vi "HapticSTM_Feedblackless_testdata.vi"() -> ()   [LabVIEW 2017]
uses:
  <userlib>/HapticSTM/Feedbackless - Testdata/Project/feedbackless.lvproj/HapticSTM.lvlib
  <userlib>/HapticSTM/Feedbackless - Testdata/Project/feedbackless.lvproj/GlobalClicksHeight.vi
  <vilib>/ptbypt/NI_PtbyPt.lvlib
  <vilib>/Utility/file.llb/Read Delimited Spreadsheet (DBL).vi
  <vilib>/Analysis/3filter.llb/Filter Passband Type.ctl
  <vilib>/Analysis/NI_AALBase.lvlib
panel:
  in  "Force Mode":u16(ring) items=["Stacked Logs", "Simple Log", "Linear"]
  out "Button":bool
  out "Zpos":cluster{dbl, "Y":dbl, i16}(graph)
  out "Filtered Current":dbl
  in  "Reset Clicks":bool
  out "Scaled Force and Current":cluster{dbl, "Filtered x":dbl, dbl}(graph)
  in  "Maximum (pA)":dbl=9000.0
  in  "Setpoint (pA)":dbl=100.0
  out "PLANE HEIGHT":dbl
  out "Current":dbl
  out "Origin Y":dbl
  out "Origin X":dbl
  out "Output Z":dbl
  in  "Rough adjust":dbl
  out "Nano Z":dbl
  out "Width":dbl
  out "VY":dbl
  out "VZ":dbl
  out "VX":dbl
  in  "Drag":dbl=1.0
  in  "STOP":bool
  in  "START":bool
  out "Fy":dbl
  out "Fz":dbl
  out "phi":dbl
  out "psi":dbl
  out "Fx":dbl
  out "theta":dbl
  out "x":dbl
  out "y":dbl
  out "z":dbl
  in  "Fine adjust":dbl=3.5
  out "Clicks":dbl
  out "Height":dbl
  # "Sample Window"
  # "Position"
  # "Sensitivity"
  # "Force"
  # "STM I/O"
  # "Angles"
  # "Current"
  # "Velocity"
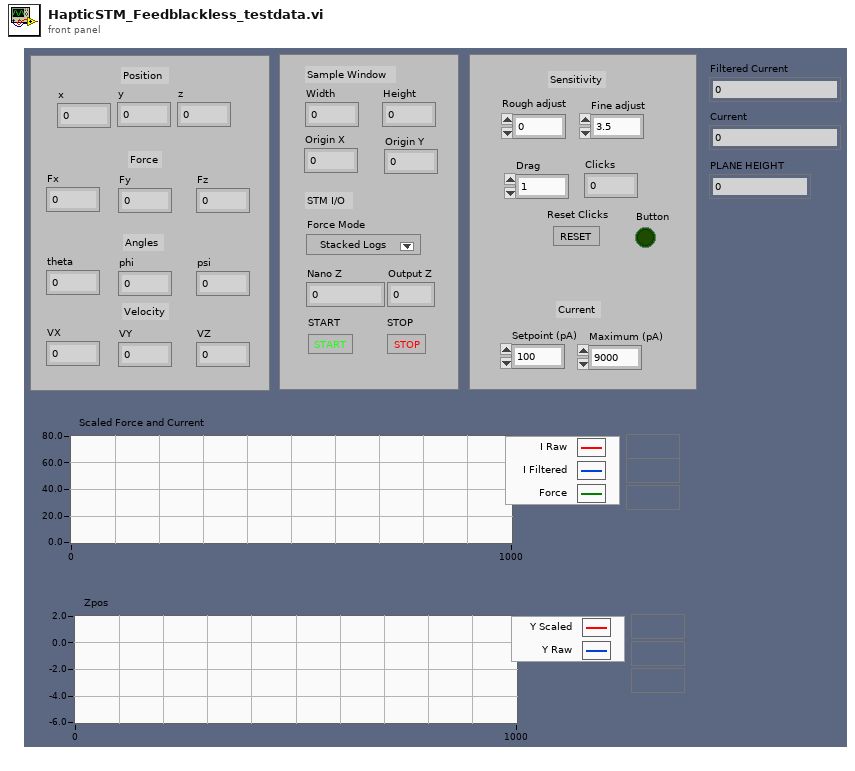
[diagram p1: front panel]
types:
  T1 = typedef "NI_AALBase.lvlib/Filter Passband Type.ctl" = enum32{"Lowpass", "Highpass", "Bandpass", "Bandstop"}
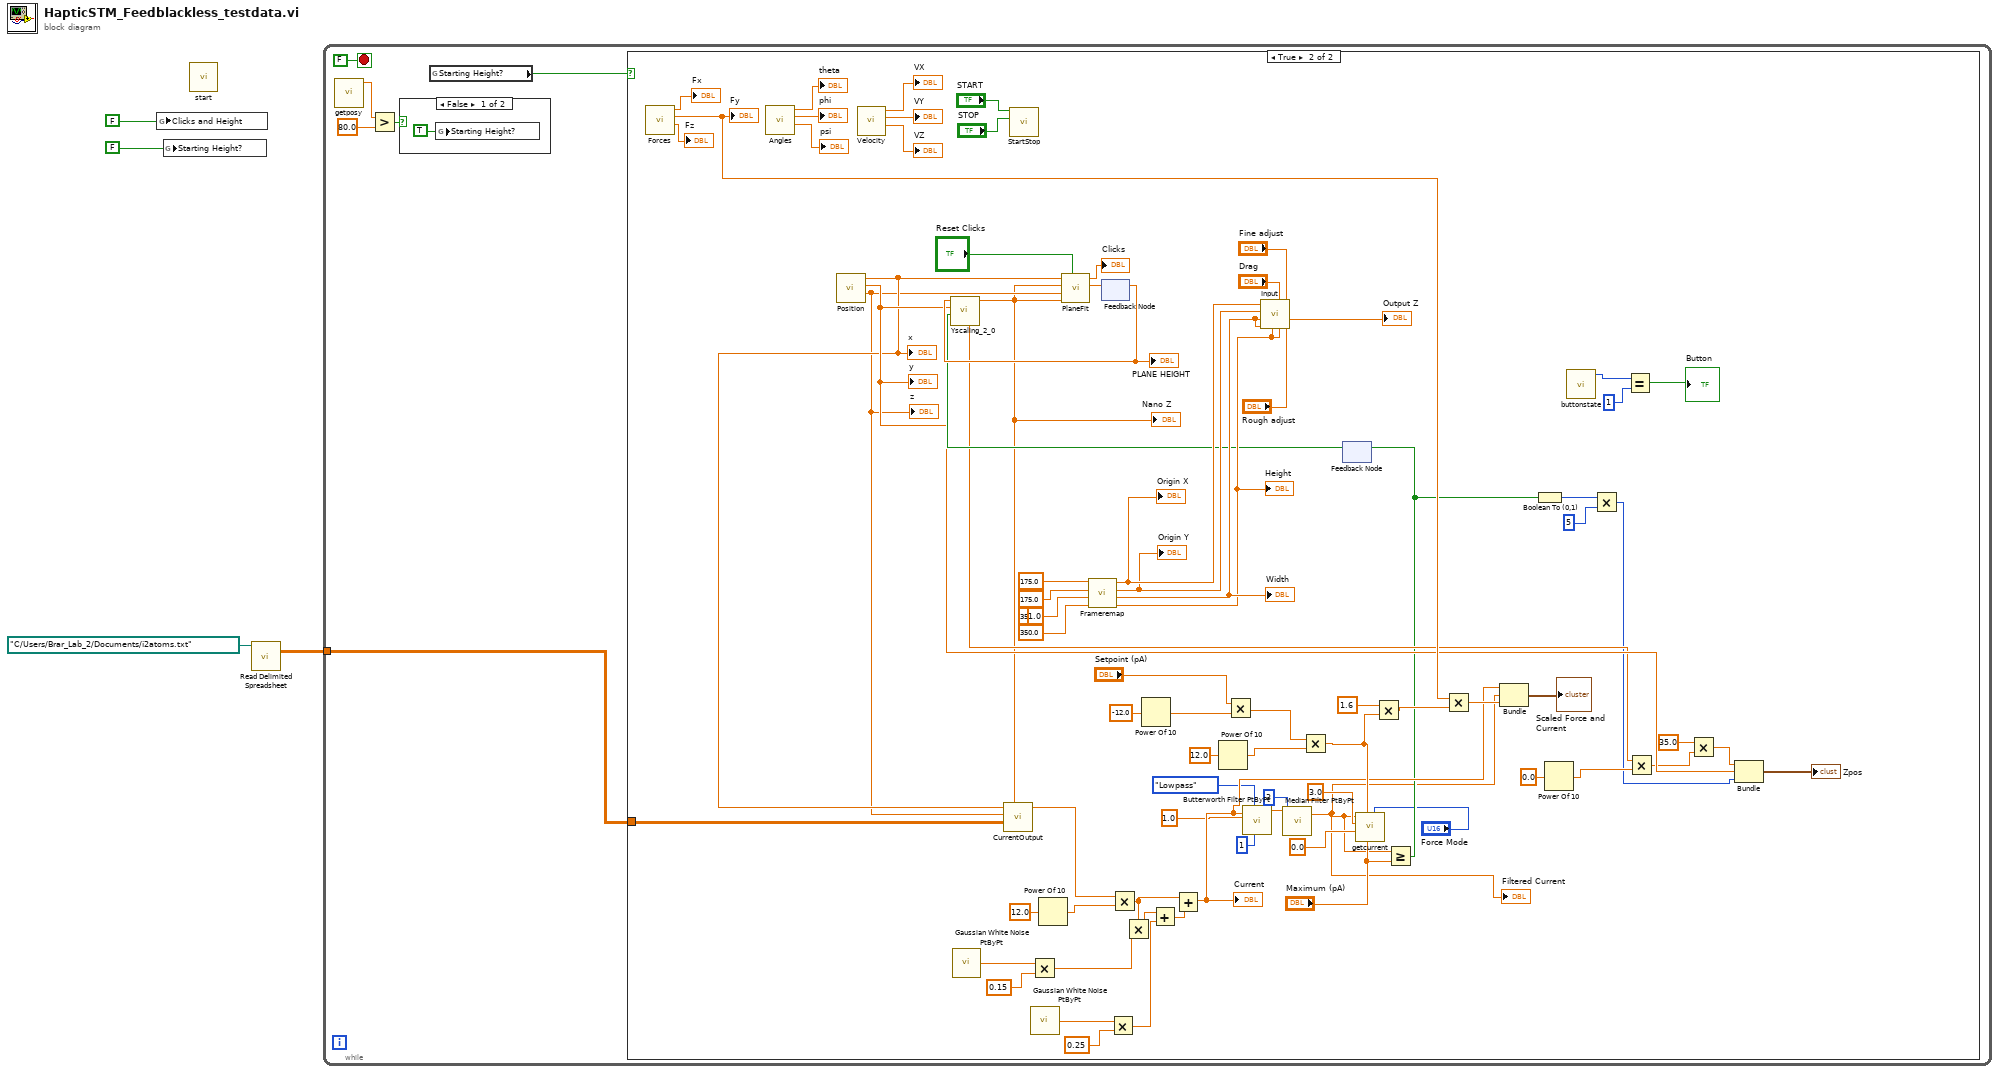
[diagram p0: block diagram]
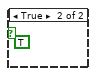
[diagram p2: hidden frame]
diagram:
  n1 = global write "GlobalClicksHeight.vi" "Clicks and Height"(FALSE ("Clicks and Height")) -> ()
  n2 = global write "GlobalClicksHeight.vi" "Starting Height?"(FALSE ("Clicks and Height")) -> ()
  n3 = call <userlib>:"start.vi"() -> ()  [unwired: 11 in, 1 out]
  n4 = call-poly <vilib>:"Read Delimited Spreadsheet.vi"("file path (dialog if empty)"=path "C:/Users/Brar_Lab_2/Documents/i2atoms.txt") -> ("all rows"=w4:dbl[][])  [unwired: 9 in, 5 out]
  n5 = while {
    tunnel: w4 -> [w10]
    stop <- FALSE stop-if-true
    n6 = call <userlib>:"getposy.vi"() -> ("function return"=w9:dbl)  [unwired: 11 in]
    n7 = Greater?(x=w9, y=80.0) -> (0:w7:bool)
    n8 = case shown="False" w7 {
      frame False {
        n9 = global write "GlobalClicksHeight.vi" "Starting Height?"(TRUE ("Starting Height?")) -> ()
      }
      frame True {
        (unwired) TRUE ("Clicks and Height")
      }
    }
    n10 = global read "GlobalClicksHeight.vi" "Starting Height?"() -> (w6:bool)
    n11 = case shown="True" w6 {
      tunnel: w10 -> [_ w13]
      frame False {
      }
      frame True {
        (unwired) 1.0 ("FO X")
        n12 = call <userlib>:"Forces.vi"() -> ("Fz"=→"Fz":dbl, "Fy"=w54:dbl, "Fx"=→"Fx":dbl)  [unwired: 9 in]
        "Fy" <- w54
        n13 = call <userlib>:"Angles.vi"() -> ("psi"=→"psi":dbl, "phi"=→"phi":dbl, "theta"=→"theta":dbl)  [unwired: 9 in]
        n14 = call <userlib>:"Position.vi"() -> ("Z"=w14:dbl, "Y"=w36:dbl, "X"=w15:dbl)  [unwired: 9 in]
        "x" <- w15
        "y" <- w36
        "z" <- w14
        n15 = call <userlib>:"Velocity.vi"() -> ("VZ"=→"VZ":dbl, "VY"=→"VY":dbl, "VX"=→"VX":dbl)  [unwired: 9 in]
        n16 = call <vilib>:"Gaussian White Noise PtByPt.vi"() -> ("Gaussian white noise"=w53:dbl)  [unwired: 3 in]
        n17 = call <userlib>:"StartStop.vi"("STOP"="STOP", "START"="START") -> ()  [unwired: 10 in]
        n18 = Multiply(x=w53, y=0.15) -> (x*y=w51:dbl)
        n19 = call <vilib>:"Gaussian White Noise PtByPt.vi"() -> ("Gaussian white noise"=w48:dbl)  [unwired: 3 in]
        n20 = Power Of 10(x=12.0) -> (10^x=w72:dbl)
        n21 = call <userlib>:"Frameremap.vi"("FH"=350.0 ("FO X"), "FW"=350.0 ("FO X"), "FO Z"=175.0 ("FO X"), "FO X"=175.0) -> ("FH"=w79:dbl, "FW"=w80:dbl, "Z Origin"=w64:dbl, "X Origin"=w65:dbl)  [unwired: 4 in]
        "Height" <- w79
        "Width" <- w80
        "Origin X" <- w65
        "Origin Y" <- w64
        n22 = feedback #1() -> (w66:dbl)  [unwired: 1 in]
        "PLANE HEIGHT" <- w66
        n23 = Multiply(x=w48, y=0.25) -> (x*y=w44:dbl)
        n24 = Power Of 10(x=-12.0) -> (10^x=w61:dbl)
        n25 = Power Of 10(x=12.0) -> (10^x=w63:dbl)
        n26 = Multiply(x="Setpoint (pA)", y=w61) -> (x*y=w59:dbl)
        n27 = call <userlib>:"Input.vi"("Current * 10^input"="Rough adjust", "Sensitivity"="Fine adjust", "Scopez"=w79, "Drag"="Drag", "FH"=w79, "FW"=w80, "Scopex"=w80, "Z origin"=w64, "X origin"=w65) -> ("Scaled Current"=→"Output Z":dbl)  [unwired: 2 in]
        n28 = Multiply(x=w59, y=w63) -> (x*y=w41:dbl)
        n29 = feedback #2() -> (w57:bool)  [unwired: 1 in]
        n30 = call <userlib>:"Yscaling_2_0.vi"("Current Maxed?"=w57, "Y"=w36, "Plane Height"=w66) -> ("y scaled"=w12:dbl, "Testoutput"=w32:dbl)  [unwired: 7 in]
        "Nano Z" <- w12
        n31 = call <userlib>:"CurrentOutput.vi"("y scaled"=w12, "array"=w13, "Z Input"=w14, "X Input"=w15) -> ("Current Out"=w16:dbl)  [unwired: 7 in]
        n32 = call <userlib>:"PlaneFit.vi"("Reset Clicks"="Reset Clicks", "Y PEN"=w12, "Z"=w14, "Nano Z"=w12, "X"=w15) -> ("Plane Height (m)"=w75:dbl, "Clicks"=→"Clicks":dbl)  [unwired: 5 in]
        n33 = feedback-in #1(w75) -> ()
        n34 = Multiply(x=w16, y=w72) -> (x*y=w50:dbl)
        n35 = Multiply(x=w50, y=w51) -> (x*y=w45:dbl)
        n36 = Add(x=w45, y=w44) -> (x+y=w46:dbl)
        n37 = Add(x=w50, y=w46) -> (x+y=w28:dbl)
        "Current" <- w28
        n38 = call <vilib>:"Butterworth Filter PtByPt.vi"("order"=1, "filter type"=Filter_Passband_Type."Lowpass", "sampling freq: fs"=1.0, "x"=w28) -> ("Filtered x"=w20:dbl)  [unwired: 5 in, 1 out]
        n39 = call <vilib>:"Median Filter PtByPt.vi"("rank"=3, "x"=w20) -> ("Filtered x"=w19:dbl)  [unwired: 2 in, 1 out]
        "Filtered Current" <- w19
        n40 = call <userlib>:"getcurrent.vi"("forcemode"="Force Mode", "maxcurrentin"="Maximum (pA)", "setpoint"=w41, "minforcey"=0.0, "maxforcey"=3.0, "currentin"=w19) -> ()  [unwired: 6 in]
        n41 = Multiply(x=1.6 ("y"), y=w41) -> (x*y=w42:dbl)
        n42 = Greater Or Equal?(x=w19, y="Maximum (pA)") -> (x >= y?=w25:bool)
        n43 = feedback-in #2(w25) -> ()
        n44 = Multiply(x=w54, y=w42) -> (x*y=w49:dbl)
        n45 = Bundle(w28, "Filtered x"=w19, w49) -> (→"Scaled Force and Current":cluster{dbl, "Filtered x":dbl, dbl})  [unwired: 1 in]
        n46 = Boolean To (0,1)(Boolean=w25) -> (0, 1=w24:i16)
        n47 = Power Of 10(x=0.0) -> (10^x=w39:dbl)
        n48 = call <userlib>:"buttonstate.vi"() -> ("function return"=w31:i32)  [unwired: 11 in]
        n49 = Multiply(x=w24, y=i16 5) -> (x*y=w22:i16)
        n50 = Equal?(x=w31, y=1) -> (x = y?=→"Button":bool)
        n51 = Multiply(x=w32, y=w39) -> (x*y=w34:dbl)
        n52 = Multiply(x=35.0, y=w34) -> (x*y=w35:dbl)
        n53 = Bundle(w35, "Y"=w36, w22) -> (→"Zpos":cluster{dbl, "Y":dbl, i16})  [unwired: 1 in]
      }
    }
  }
